vi "Tilt range alarm.vi"(1 "Radius":dbl=5.0, 2 "Y-Stored":dbl, 3 "X-Stored":dbl, 4 "Y-Actual":dbl, 5 "X-Actual":dbl) -> (0 "Alarm":bool)   [LabVIEW 2019]
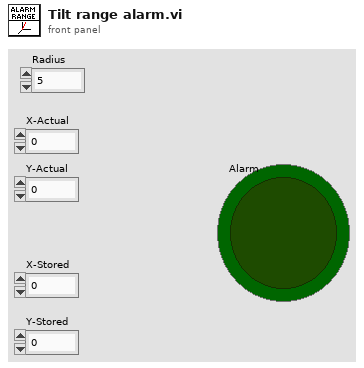
[diagram p1: front panel]
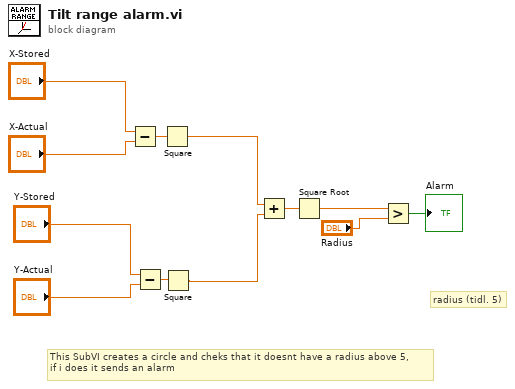
[diagram p0: block diagram]
diagram:
  # "radius (tidl. 5)"
  # "This SubVI creates a circle and cheks that it doesnt have a radius above 5,\nif i does it sends an alarm"
  n1 = Subtract(x="X-Stored", y="X-Actual") -> (x-y=w5:dbl)
  n2 = Subtract(x="Y-Stored", y="Y-Actual") -> (x-y=w7:dbl)
  n3 = Square(x=w5) -> (x^2=w4:dbl)
  n4 = Square(x=w7) -> (x^2=w6:dbl)
  n5 = Add(x=w4, y=w6) -> (x+y=w3:dbl)
  n6 = Square Root(x=w3) -> (sqrt(x)=w2:dbl)
  n7 = Greater?(x=w2, y="Radius") -> (0:→"Alarm":bool)
